vi "SF2 Start Stop Recording.vi"(11 "Record":bool) -> ()   [LabVIEW 2016]
uses:
  _Notifier/SF2_ActionTypeDef.ctl
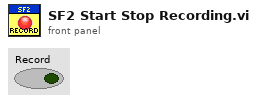
[diagram p1: front panel]
types:
  T1 = typedef "SF2_ActionTypeDef.ctl" = enum16{"None", "Halt", "Start Recording", "Stop Recording", "Reset Buffer"}
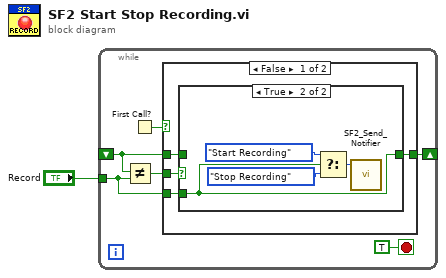
[diagram p0: block diagram]
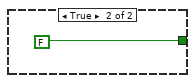
[diagram p3: hidden frame]
diagram:
  n1 = while {
    shift-right: [w6] -> _
    shift-left: _ -> [w5]
    tunnel: "Record" -> [w2]
    stop <- TRUE stop-if-true
    n2 = Not Equal?(x=w5, y=w2) -> (x != y?=w4:bool)
    n3 = First Call?() -> (First Call?: T/F=w3:bool)
    n4 = case shown="False" w3 {
      tunnel: [w11 FALSE] -> w6
      tunnel: w5 -> [w10 _]
      tunnel: w4 -> [w9 _]
      tunnel: w2 -> [w8 _]
      frame False {
        n5 = case shown="True" w9 {
          tunnel: [w12 w16] -> w11
          tunnel: w10 -> [w12 _]
          tunnel: w8 -> [_ w16]
          frame False {
          }
          frame True {
            n6 = Select(t=SF2_ActionTypeDef."Start Recording" ("SF2 Action"), s=w16, f=SF2_ActionTypeDef."Stop Recording" ("SF2 Action")) -> (s? t:f=w13:T1)
            n7 = call "SF2_Send_Notifier.vi"("SF2 Action"=w13) -> ()  [unwired: 11 in]
          }
        }
      }
      frame True {
      }
    }
  }
